vi "from string.vi"(8 "error in":errorcluster, 9 "data":string, 10 "version":string, 11 "DMM configuration in":refnum<class "DMM configuration.lvclass">) -> (0 "error out":errorcluster, 3 "DMM configuration out":refnum<class "DMM configuration.lvclass">)   [LabVIEW 2025, in "DMM.lvlib" / "DMM configuration.lvclass"]
doc: "Provides an interface for loading a module configuration from a file or other serialized data source. It is recommended that all children of this class store data in two sets--data required for its own initialization, and any data required for parent initialization--and that each implementation uses the <b>Call Parent Method</b> primitive to de-serialize parent information.Copyright 2017 National Instruments Corporation\n\nLicensed under the Apache License, Version 2.0 (the \"License\"); you may not use this file except in compliance with the License. You may obtain a copy of the License at http://www.apache.org/licenses/LICENSE-2.0\nUnless required by applicable law or agreed to in writing, software distributed under the License is distributed on an \"AS IS\" BASIS, WITHOUT WARRANTIES OR CONDITIONS OF ANY KIND, either express or implied. See the License for the specific language governing permissions and limitations under the License."
uses:
  DMM configuration.lvclass
  DMM Setting.ctl
  DMM configuration.lvclass/DMM configuration.ctl
  Users/Public/Documents/Sandia National Labs/TSS Plugin/Abstract Engine.lvlibp/Plugin/Abstract/Instrument configuration/Instrument configuration.lvclass
  Users/Public/Documents/Sandia National Labs/TSS Plugin/CEF.lvlibp/serializable configuration/CEF_serializable configuration.lvclass
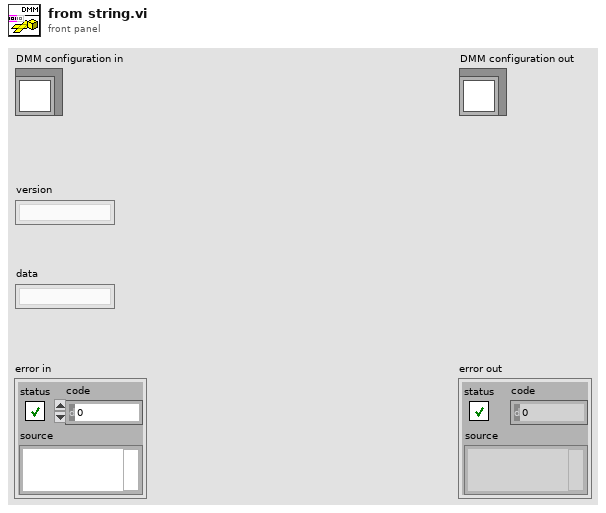
[diagram p1: front panel]
types:
  T1 = typedef "DMM.lvlib/DMM configuration.lvclass/DMM Setting.ctl" = cluster{"Function":string, "CurrentSource":string, "Resolution":string, "Range":dbl}
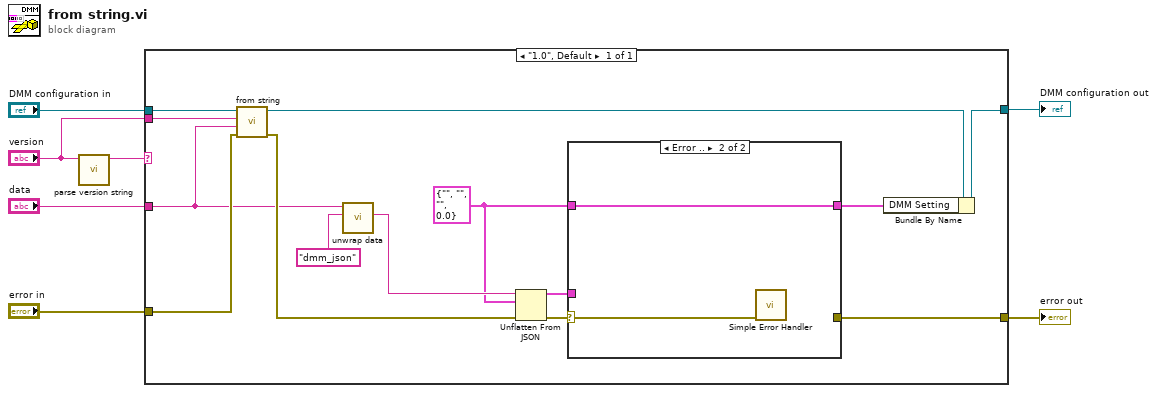
[diagram p0: block diagram]
diagram:
  n1 = call "parse version string.vi"("full version"="version") -> ("major.minor version"=w3:string)  [unwired: 7 in, 3 out]
  n2 = case shown="\"1.0\", Default" w3 {
    tunnel: "DMM configuration in" -> [w21]
    tunnel: [w15] -> w6
    tunnel: "data" -> [w13]
    tunnel: "error in" -> [w19]
    tunnel: "version" -> [w14]
    tunnel: [w11] -> w1
    frame "1.0", Default {
      w9 = T1 {"Function"="", "CurrentSource"="", "Resolution"="", "Range"=0.0} ("Setting")
      n3 = call-parent "from string.vi"("error in"=w19, "data"=w13, "version"=w14, "Instrument configuration"=w21) -> ("error out"=w18:errorcluster, "Instrument configuration out"=w16:refnum<class "DMM configuration.lvclass">)  [unwired: 6 in]
      n4 = call "unwrap data.vi"("identifier"="dmm_json" ("additional identifier"), "data to unwrap"=w13) -> ("unwrapped data"=w17:string)  [unwired: 8 in, 1 out]
      n5 = Unflatten From JSON(JSON string=w17, type and defaults=w9, error in (no error)=w18) -> (value=w10:T1, error out=w12:errorcluster)  [unwired: 4 in]
      n6 = case shown="Error .." w12 {
        selector: w12 -> [w22 w25]
        tunnel: w10 -> [w23 _]
        tunnel: [w23 w24] -> w8
        tunnel: w9 -> [_ w24]
        tunnel: [w22 _] -> w11
        frame No Error {
        }
        frame Error {
          n7 = call <vilib>:"Simple Error Handler.vi"("error in (no error)"=w25) -> ()  [unwired: 4 in, 5 out]
        }
      }
      n8 = Bundle By Name(cluster=w16, "DMM Setting"=w8) -> (w15:refnum<class "DMM configuration.lvclass">)
    }
  }
  "error out" <- w1
  "DMM configuration out" <- w6
